vi "保存程序.vi"(8 "error in (no error)":errorcluster caption="错误输入（无错误）", 11 "程序 输入":refnum<class "程序.lvclass">) -> (0 "error out":errorcluster caption="错误输出", 3 "程序 输出":refnum<class "程序.lvclass">)   [LabVIEW 2018, in "程序.lvclass"]
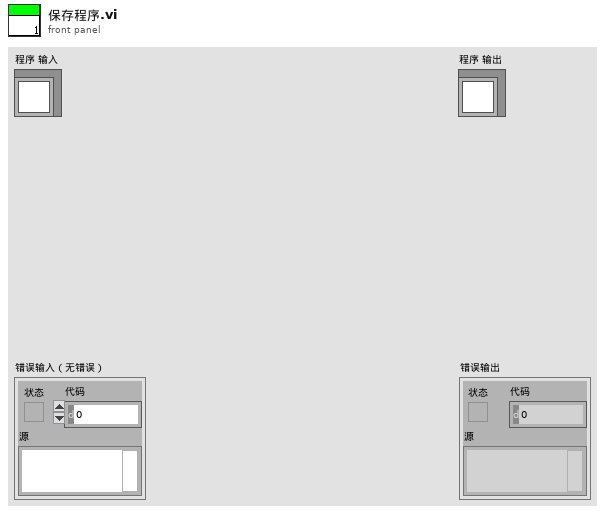
[diagram p1: front panel]
types:
  T1 = enum16{"open", "replace", "create", "open or create", "replace or create", "replace or create with confirmation"}
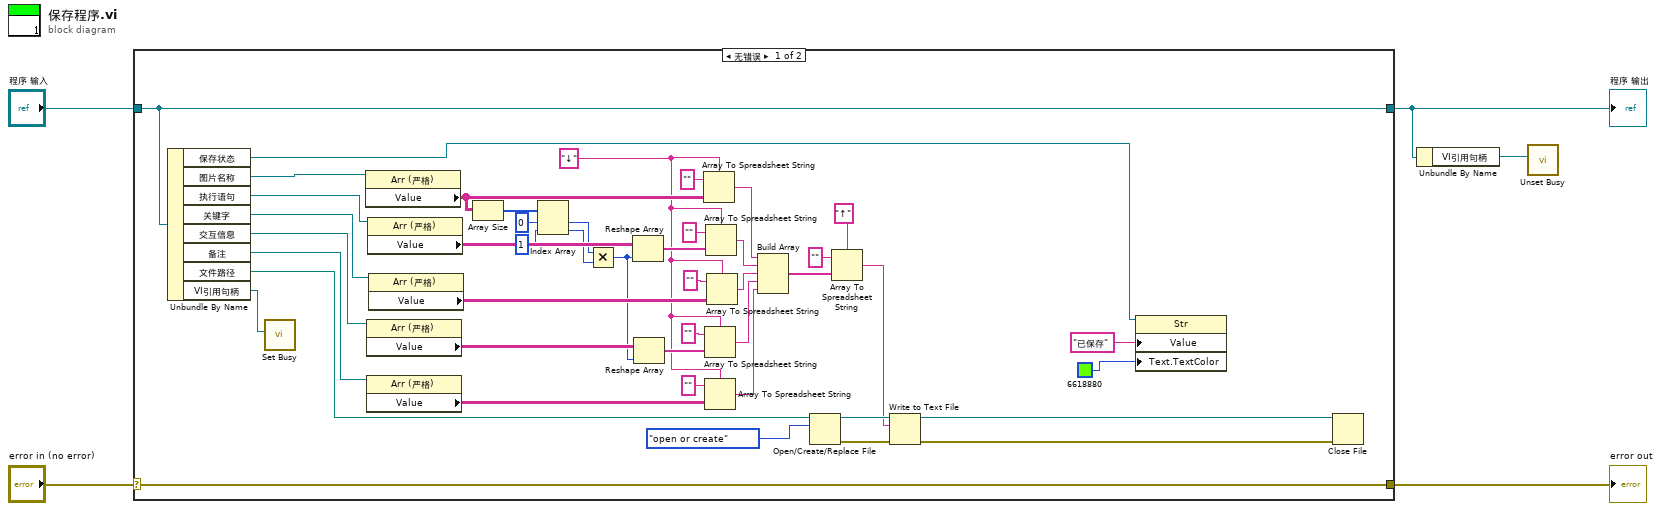
[diagram p0: block diagram]
diagram:
  n1 = case shown="无错误" "error in (no error)" {
    selector: "error in (no error)" -> [w50 w52]
    tunnel: [w50 w52] -> w4
    tunnel: [w42 w51] -> w2
    tunnel: "程序 输入" -> [w42 w51]
    frame No Error {
      w11 = "↓" ("分隔符(Tab)")
      n2 = Unbundle By Name(w42) -> ("保存状态"=w8:refnum<vi>, "图片名称"=w41:refnum<vi>, "执行语句"=w40:refnum<vi>, "关键字"=w39:refnum<vi>, "交互信息"=w27:refnum<vi>, "备注"=w14:refnum<vi>, "文件路径"=w30:path, "VI引用句柄"=w6:refnum<vi>)
      n3 = call <vilib>:"Set Busy.vi"("VI reference (current VI)"=w6) -> ()  [unwired: 9 in, 2 out]
      n4 = property class="Arr (严格)"(reference=w41) -> ("Value"=w21:string[][])  [unwired: 1 in, 2 out]
      n5 = property class="Arr (严格)"(reference=w27) -> ("Value"=w25:string[][])  [unwired: 1 in, 2 out]
      n6 = property class="Arr (严格)"(reference=w14) -> ("Value"=w13:string[][])  [unwired: 1 in, 2 out]
      n7 = property class="Arr (严格)"(reference=w40) -> ("Value"=w23:string[][])  [unwired: 1 in, 2 out]
      n8 = property class="Arr (严格)"(reference=w39) -> ("Value"=w35:string[][])  [unwired: 1 in, 2 out]
      n9 = Array Size(array=w21) -> (size(s)=w20:i32[])
      n10 = Index Array(array=w20, index #1=0 ("索引"), index #2=1 ("索引")) -> (element #1=w17:i32, element #2=w16:i32)
      n11 = Multiply(x=w17, y=w16) -> (x*y=w15:i32)
      n12 = Reshape Array(w23, w15) -> (w22:string[])
      n13 = Reshape Array(w25, w15) -> (w24:string[])
      n14 = Array To Spreadsheet String(delimiter (Tab)=w11, array=w21, 3:"" ("格式字符串")) -> (spreadsheet string=w34:string)
      n15 = Array To Spreadsheet String(delimiter (Tab)=w11, array=w24, 3:"" ("格式字符串")) -> (spreadsheet string=w26:string)
      n16 = Array To Spreadsheet String(delimiter (Tab)=w11, array=w13, 3:"" ("格式字符串")) -> (spreadsheet string=w10:string)
      n17 = Array To Spreadsheet String(delimiter (Tab)=w11, array=w22, 3:"" ("格式字符串")) -> (spreadsheet string=w33:string)
      n18 = Array To Spreadsheet String(delimiter (Tab)=w11, array=w35, 3:"" ("格式字符串")) -> (spreadsheet string=w32:string)
      n19 = Build Array(w34, w33, w32, w26, w10) -> (w31:string[])
      n20 = Open/Create/Replace File(file path (use dialog)=w30, operation (0:open)=T1."open or create" ("操作(0:open)")) -> (refnum out=w49:refnum<file>, error out=w48:errorcluster)  [unwired: 4 in, 1 out]
      n21 = Array To Spreadsheet String(delimiter (Tab)="↑" ("分隔符(Tab)"), array=w31, 3:"" ("格式字符串")) -> (spreadsheet string=w44:string)
      n22 = Write to Text File(file (use dialog)=w49, text=w44, error in=w48) -> (refnum out=w47:refnum<file>, error out=w46:errorcluster)  [unwired: 1 in, 1 out]
      n23 = property class="Str"(reference=w8, "Value"="已保存" ("值"), "Text.TextColor"=u32 6618880) -> ()  [unwired: 1 in, 2 out]
      n24 = Close File(refnum=w47, error in=w46) -> ()  [unwired: 2 out]
    }
    frame Error {
    }
  }
  "error out" <- w4
  "程序 输出" <- w2
  n25 = Unbundle By Name(w2) -> ("VI引用句柄"=w1:refnum<vi>)
  n26 = call <vilib>:"Unset Busy.vi"("VI reference (current VI)"=w1) -> ()  [unwired: 10 in, 1 out]
